vi "GetType.vi"(8 "error in (no error)":errorcluster, 11 "CS++PVUpdate Msg in":refnum<class "CS++PVUpdate Msg.lvclass">) -> (0 "error out":errorcluster, 2 "Data Sample":variant, 3 "CS++PVUpdate Msg out":refnum<class "CS++PVUpdate Msg.lvclass">)   [LabVIEW 2014, in "CS++PVMonitor.lvlib" / "CS++PVUpdate Msg.lvclass"]
doc: "This VI delivers a sample of the data type format the message expects."
uses:
  CS++PVUpdate Msg.lvclass
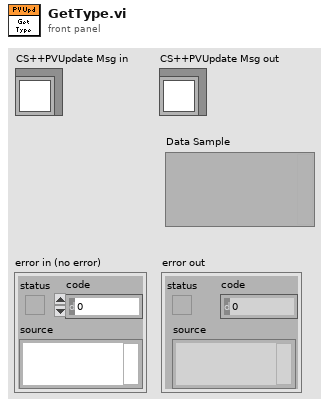
[diagram p1: front panel]
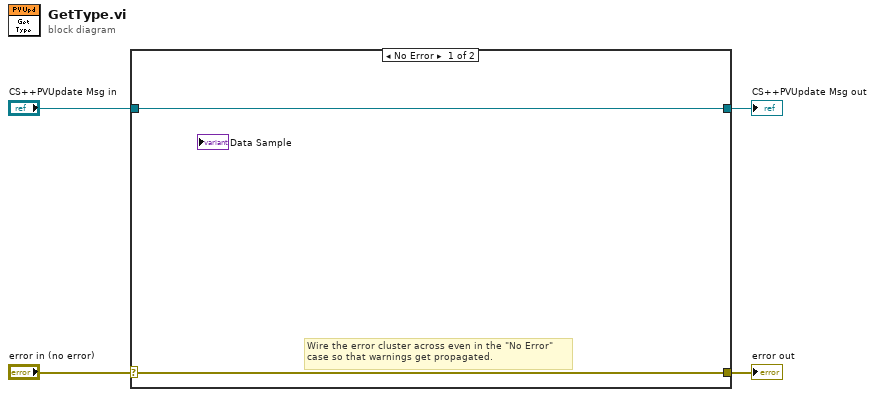
[diagram p0: block diagram]
diagram:
  n1 = case shown="No Error" "error in (no error)" {
    selector: "error in (no error)" -> [w5 w8]
    tunnel: [w5 w8] -> w3
    tunnel: [w6 w7] -> w1
    tunnel: "CS++PVUpdate Msg in" -> [w6 w7]
    frame No Error {
      # "Wire the error cluster across even in the \"No Error\"\ncase so that warnings get propagated."
    }
    frame Error {
    }
  }
  "error out" <- w3
  "CS++PVUpdate Msg out" <- w1
